vi "Alp Seq Put.vi"(6 "UserArrayPtr":u8[](array[numeric])=array[4097 elements], 7 "PicLoad":i32, 8 "error in (no error)":errorcluster, 9 "PicOffset":i32, 10 "SequenceId":u32, 11 "DeviceId":u32) -> (0 "error out":errorcluster, 3 "function return":i32, 4 "UserArrayPtr out":u8[](array[numeric]))   [LabVIEW 2013, in "alpD41.lvlib"]
uses:
  alpD41.lvlib
  alpD41.dll
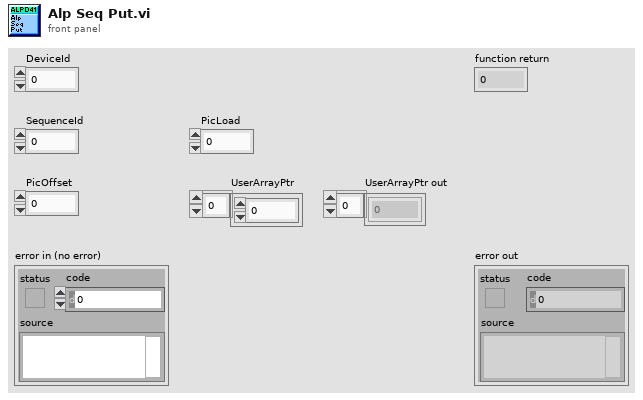
[diagram p1: front panel]
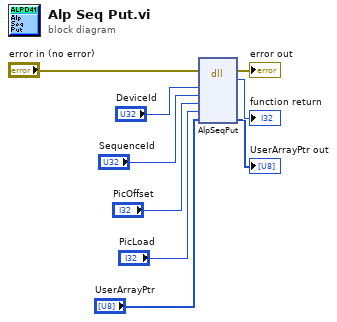
[diagram p0: block diagram]
diagram:
  n1 = dll-call lib="C:/Users/ErNa/Google Drive (ernajqi@gmail.com)/ErNa/LabView/DMD Standalone Codes/Libraries-alpD41/alpD41.*" fn="AlpSeqPut"(error in="error in (no error)", "DeviceId"="DeviceId", "SequenceId"="SequenceId", "PicOffset"="PicOffset", "PicLoad"="PicLoad", "UserArrayPtr"="UserArrayPtr") -> (error out=→"error out":errorcluster, →"function return":i32, "UserArrayPtr"=→"UserArrayPtr out":u8[])  [unwired: 6 in, 1 out]
